vi "AO Close.vi"(8 "error in (no error)":errorcluster, 11 "FC2901 in":refnum<class "FC2901.lvclass">) -> (0 "error out":errorcluster)   [LabVIEW 2021, in "FC2901.lvclass"]
uses:
  FC2901.lvclass
  FC2901.lvclass/FC2901.ctl
  <vilib>/NathanCo/Analog-Tasks/Analog Output/Analog Output/Analog Output.lvclass
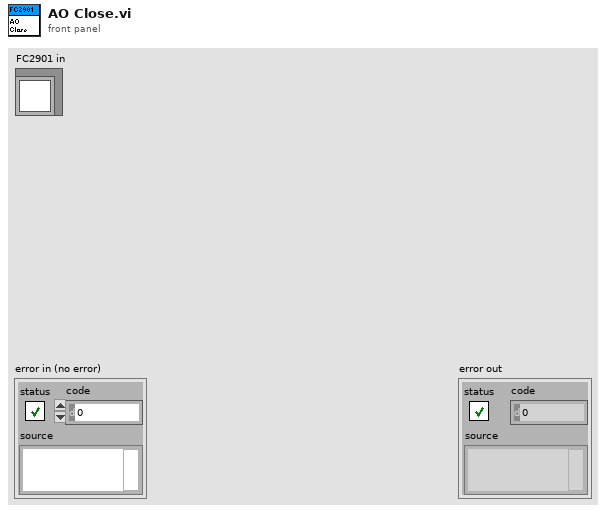
[diagram p1: front panel]
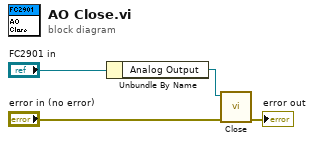
[diagram p0: block diagram]
diagram:
  n1 = Unbundle By Name("FC2901 in") -> ("Analog Output"=w3:refnum<class "Analog Output.lvclass">)
  n2 = call <vilib>:"Close.vi"("error in (no error)"="error in (no error)", "Analog Output in"=w3) -> ("error out"=→"error out":errorcluster)  [unwired: 9 in]
